vi "Flat seque for 2nd machin.vi"(0 "Сщечик брака":i32, 1 "Defect":bool, 3 "Ускоренно/Реально":bool, 5 "Время до коробки (с)":i32, 7 "Время между станками (с)":i32, 9 "Время до урны (с)":i32, 11 "Время на обработку (с)":i32, 12 "Время загрузки\n второго станка (с)":i32) -> (4 "Брак":i32)   [LabVIEW 2020]
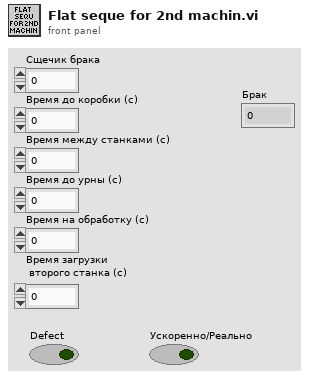
[diagram p1: front panel]
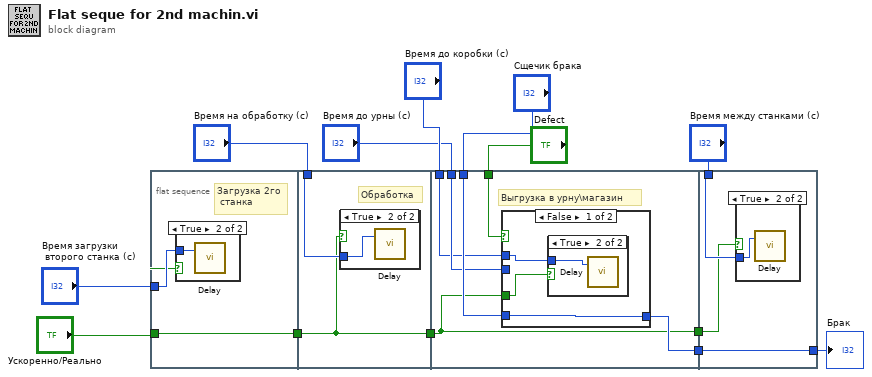
[diagram p0: block diagram]
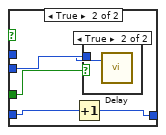
[diagram p5: hidden frame]
diagram:
  n1 = flat-sequence {
    tunnel: "Время загрузки\n второго станка (с)" -> [w15]
    tunnel: "Ускоренно/Реально" -> [w14]
    tunnel: [w14] -> w13
    tunnel: "Время на обработку (с)" -> [w18]
    tunnel: w13 -> [w17]
    tunnel: [w17] -> w12
    tunnel: "Defect" -> [w25]
    tunnel: "Сщечик брака" -> [w24]
    tunnel: "Время до урны (с)" -> [w23]
    tunnel: "Время до коробки (с)" -> [w22]
    tunnel: [w21] -> w11
    tunnel: w12 -> [w20]
    tunnel: [w20] -> w10
    tunnel: [w37] -> w1
    tunnel: w11 -> [w37]
    tunnel: "Время между станками (с)" -> [w36]
    tunnel: w10 -> [w35]
    frame #0 {
      # "Загрузка 2го\n станка"
      n2 = case shown="True" w14 {
        tunnel: w15 -> [_ w16]
        frame False {
        }
        frame True {
          n3 = call "Delay.vi"("Wait (s)"=w16) -> ()  [unwired: 1 in, 1 out]
        }
      }
    }
    frame #1 {
      # "Обработка"
      n4 = case shown="True" w17 {
        tunnel: w18 -> [_ w19]
        frame False {
        }
        frame True {
          n5 = call "Delay.vi"("Wait (s)"=w19) -> ()  [unwired: 1 in, 1 out]
        }
      }
    }
    frame #2 {
      # "Выгрузка в урну\\магазин"
      n6 = case shown="False" w25 {
        tunnel: w24 -> [w28 w33]
        tunnel: [w28 w32] -> w21
        tunnel: w23 -> [_ w31]
        tunnel: w22 -> [w27 _]
        tunnel: w20 -> [w26 w30]
        frame False {
          n7 = case shown="True" w26 {
            tunnel: w27 -> [_ w29]
            frame False {
            }
            frame True {
              n8 = call "Delay.vi"("Wait (s)"=w29) -> ()  [unwired: 1 in, 1 out]
            }
          }
        }
        frame True {
          n9 = Increment(x=w33) -> (x+1=w32:i32)
          n10 = case shown="True" w30 {
            tunnel: w31 -> [_ w34]
            frame False {
            }
            frame True {
              n11 = call "Delay.vi"("Wait (s)"=w34) -> ()  [unwired: 1 in, 1 out]
            }
          }
        }
      }
    }
    frame #3 {
      n12 = case shown="True" w35 {
        tunnel: w36 -> [_ w38]
        frame False {
        }
        frame True {
          n13 = call "Delay.vi"("Wait (s)"=w38) -> ()  [unwired: 1 in, 1 out]
        }
      }
    }
  }
  "Брак" <- w1
